vi "LoadSimbolProperties.vi"(8 "error in (no error)":errorcluster, 10 "name":string, 11 "TCatAdsNet in":refnum<class "AdsNET.lvclass">) -> (0 "error out":errorcluster, 1 "Elements":i32, 2 "SymbolProperties":T1, 3 "TCatAdsNet out":refnum<class "AdsNET.lvclass">)   [LabVIEW 2016, in "TCatAdsNet.lvlib" / "AdsNET.lvclass"]
doc: "Call this method to obtain information about the individual symbols (variables) in ADS devices."
uses:
  AdsNET.lvclass
  AdsNET.lvclass/AdsNET.ctl
  C:/Users/Maurizio/Projects/twincat-lv-ads-library/TCatAdsNet Library/TwinCAT.Ads.dll
  TwinCAT.Ads.dll
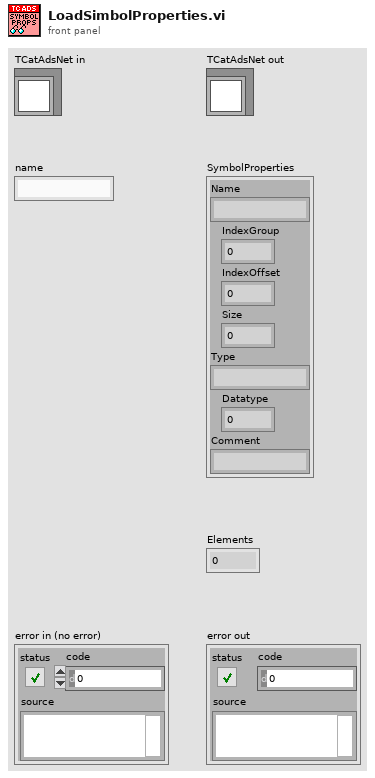
[diagram p1: front panel]
types:
  T1 = cluster{"Name":string, "IndexGroup":i64, "IndexOffset":i64, "Size":i32, "Type":string, "Datatype":i32, "Comment":string}
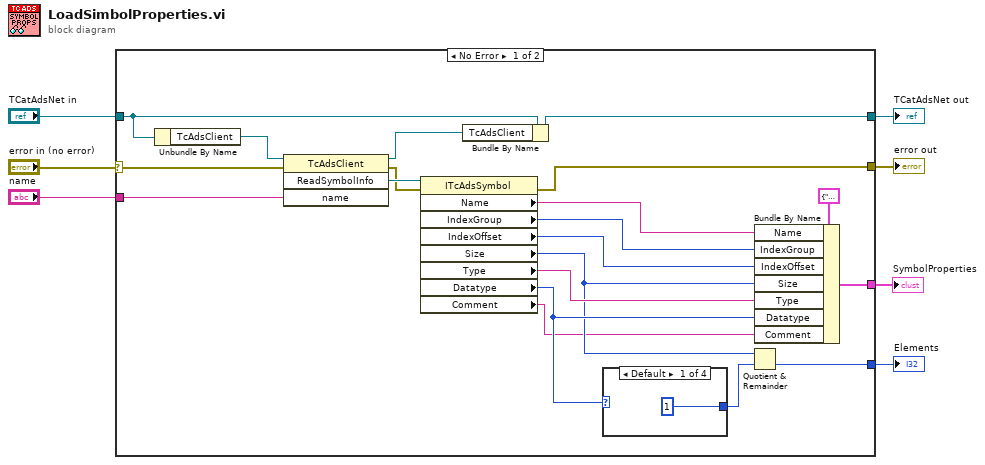
[diagram p0: block diagram]
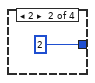
[diagram p2: hidden frame]
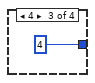
[diagram p3: hidden frame]
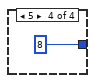
[diagram p4: hidden frame]
diagram:
  n1 = case shown="No Error" "error in (no error)" {
    selector: "error in (no error)" -> [w9 w32]
    tunnel: "TCatAdsNet in" -> [w27 w33]
    tunnel: "name" -> [w25 _]
    tunnel: [w23 w33] -> w5
    tunnel: [w20 w32] -> w4
    tunnel: [w14 _] -> w1
    tunnel: [w10 _] -> w3
    frame No Error {
      n2 = Unbundle By Name(w27) -> ("TcAdsClient"=w26:refnum<k24>)
      n3 = invoke class="TcAdsClient" method="ReadSymbolInfo"(reference=w26, error in=w9, "name"=w25) -> (reference out=w22:refnum<k24>, error out=w21:errorcluster, "ReadSymbolInfo"=w24:refnum<k24>)  [unwired: 1 in, 1 out]
      n4 = property class="ITcAdsSymbol"(reference=w24, error in=w21) -> (error out=w20:errorcluster, "Name"=w18:string, "IndexGroup"=w17:i64, "IndexOffset"=w16:i64, "Size"=w12:i32, "Type"=w15:string, "Datatype"=w13:i32, "Comment"=w8:string)  [unwired: 1 out]
      n5 = Bundle By Name(cluster=w27, "TcAdsClient"=w22) -> (w23:refnum<class "AdsNET.lvclass">)
      n6 = case shown="Default" w13 {
        tunnel: [1 2 4 8] -> w11
        frame Default {
        }
        frame 2 {
        }
        frame 4 {
        }
        frame 5 {
        }
      }
      n7 = Quotient & Remainder(x=w12, y=w11) -> (floor(x/y)=w10:i32)  [unwired: 1 out]
      n8 = Bundle By Name(cluster=T1 {"Name"="", "IndexGroup"=0, "IndexOffset"=0, "Size"=0, "Type"="", "Datatype"=0, "Comment"=""}, "Name"=w18, "IndexGroup"=w17, "IndexOffset"=w16, "Size"=w12, "Type"=w15, "Datatype"=w13, "Comment"=w8) -> (w14:T1)
    }
    frame Error {
    }
  }
  "TCatAdsNet out" <- w5
  "error out" <- w4
  "Elements" <- w3
  "SymbolProperties" <- w1
